vi "DualButton BiStateVariableToggle.vi"(8 "PreviousState":u16(ring) items=["State1", "State2"], 10 "ButtonToSelect\nSecondState":bool, 11 "ButtonToSelect\nFirstState":bool) -> (0 "NewState":u16(ring) items=["State1", "State2"])   [LabVIEW 2017]
doc: "Allows a pair of buttons to switch the value of an enumerated GlobalVariable between two possible states. One button press selects 1 state, the other button press selects the alternate state."
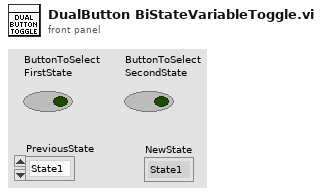
[diagram p1: front panel]
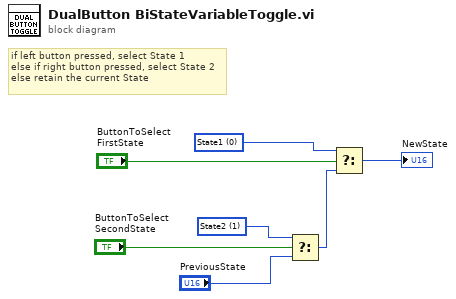
[diagram p0: block diagram]
diagram:
  w1 = u16 0 items=["State1", "State2"] ("PreviousState")
  w2 = u16 1 items=["State1", "State2"] ("PreviousState")
  # "if left button pressed, select State 1\nelse if right button pressed, select State 2\nelse retain the current State"
  n1 = Select(t=w2, s="ButtonToSelect\nSecondState", f="PreviousState") -> (s? t:f=w6:u16)
  n2 = Select(t=w1, s="ButtonToSelect\nFirstState", f=w6) -> (s? t:f=→"NewState":u16)
